vi "Model - DeInit.vi"(8 "error in (no error)":errorcluster, 11 "View Model":T1) -> (0 "error out":errorcluster)   [LabVIEW 2017]
doc: "De - initialize View Model"
uses:
  Controls/View Model.ctl
  Configuration/Controls/Config Model.ctl
  Configuration/Controls/Config Data.ctl
  Error Handler/Controls/Error Model.ctl
  Error Handler/Controls/Error Data.ctl
  Error Handler/Controls/Error Type.ctl
  Controls/Shared Model.ctl
  Elevator Controller/Controls/Elevator Model.ctl
  Elevator Controller/Controls/Elevator Location.ctl
  Elevator Controller/Controls/Elevator CMD Data.ctl
  Elevator Controller/Controls/Elevator Commands.ctl
  Elevator Controller/Controls/Elevator Overhead.ctl
  Elevator Controller/Controls/Elevator States.ctl
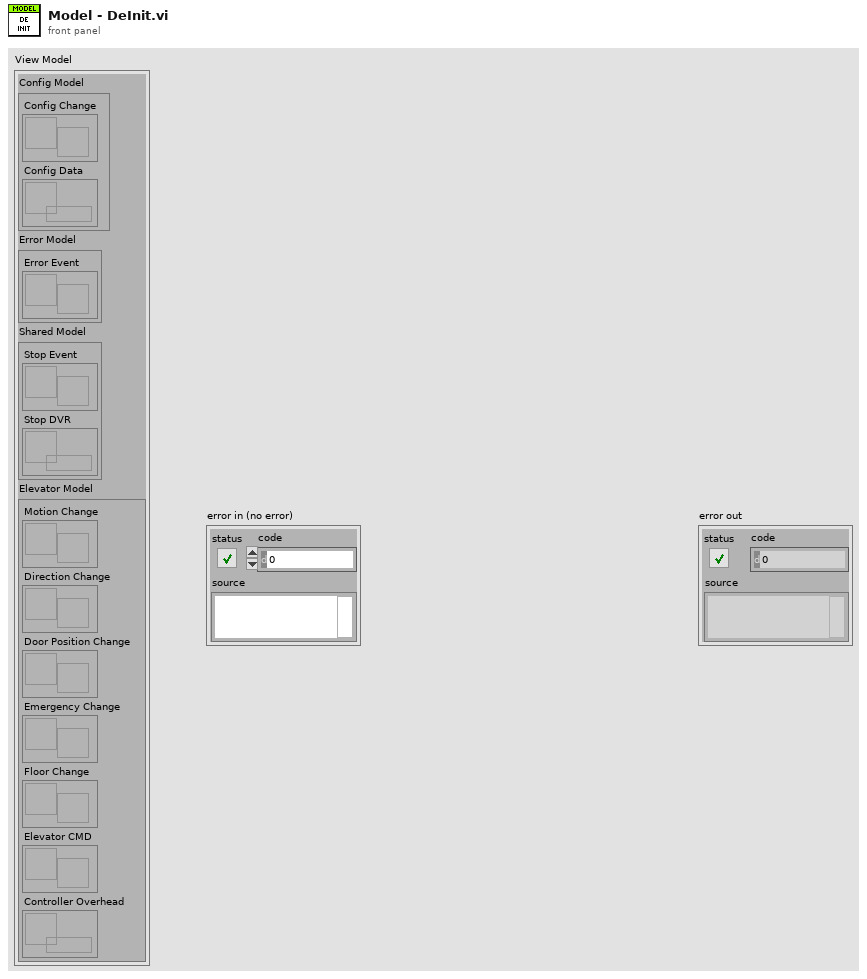
[diagram p1: front panel]
types:
  T1 = typedef "View Model.ctl" = cluster{"Config Model":T2, "Error Model":T3, "Shared Model":T4, "Elevator Model":T5}
  T2 = typedef "Config Model.ctl" = cluster{"Config Change":refnum<user-event>, "Config Data":refnum<data-value>}
  T3 = typedef "Error Model.ctl" = cluster{"Error Event":refnum<user-event>}
  T4 = typedef "Shared Model.ctl" = cluster{"Stop Event":refnum<user-event>, "Stop DVR":refnum<data-value>}
  T5 = typedef "Elevator Model.ctl" = cluster{"Motion Change":refnum<user-event>, "Direction Change":refnum<user-event>, "Door Position Change":refnum<user-event>, "Emergency Change":refnum<user-event>, "Floor Change":refnum<user-event>, "Elevator CMD":refnum<user-event>, "Controller Overhead":refnum<data-value>}
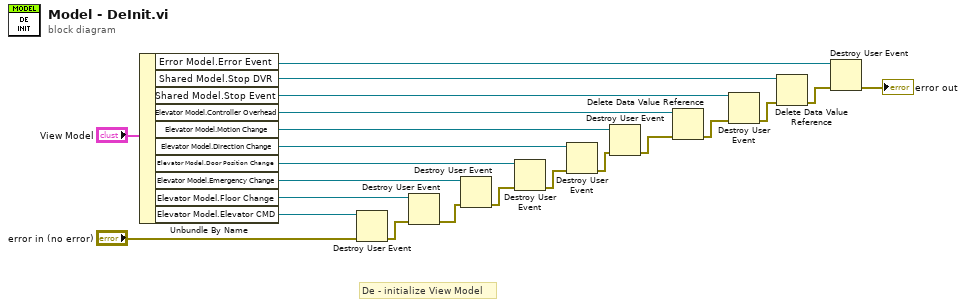
[diagram p0: block diagram]
diagram:
  # "De - initialize View Model"
  n1 = Unbundle By Name("View Model") -> ("Error Model.Error Event"=w13:refnum<user-event>, "Shared Model.Stop DVR"=w12:refnum<data-value>, "Shared Model.Stop Event"=w11:refnum<user-event>, "Elevator Model.Controller Overhead"=w10:refnum<data-value>, "Elevator Model.Motion Change"=w9:refnum<user-event>, "Elevator Model.Direction Change"=w8:refnum<user-event>, "Elevator Model.Door Position Change"=w7:refnum<user-event>, "Elevator Model.Emergency Change"=w6:refnum<user-event>, "Elevator Model.Floor Change"=w5:refnum<user-event>, "Elevator Model.Elevator CMD"=w4:refnum<user-event>)
  n2 = Destroy User Event(user event=w4, error in="error in (no error)") -> (error out=w3:errorcluster)
  n3 = Destroy User Event(user event=w5, error in=w3) -> (error out=w22:errorcluster)
  n4 = Destroy User Event(user event=w6, error in=w22) -> (error out=w21:errorcluster)
  n5 = Destroy User Event(user event=w7, error in=w21) -> (error out=w20:errorcluster)
  n6 = Destroy User Event(user event=w8, error in=w20) -> (error out=w19:errorcluster)
  n7 = Destroy User Event(user event=w9, error in=w19) -> (error out=w18:errorcluster)
  n8 = Delete Data Value Reference(data value reference=w10, error in=w18) -> (error out=w17:errorcluster)  [unwired: 1 out]
  n9 = Destroy User Event(user event=w11, error in=w17) -> (error out=w16:errorcluster)
  n10 = Delete Data Value Reference(data value reference=w12, error in=w16) -> (error out=w15:errorcluster)  [unwired: 1 out]
  n11 = Destroy User Event(user event=w13, error in=w15) -> (error out=→"error out":errorcluster)
